vi "Clean Up.vi"(8 "error in (no error)":errorcluster, 11 "PXI in":refnum<class "PXI.lvclass">) -> (0 "error out":errorcluster, 3 "PXI out":refnum<class "PXI.lvclass">)   [LabVIEW 2013, in "PXI.lvclass"]
uses:
  PXI.lvclass
  PXI.lvclass/PXI.ctl
  <resource>/objmgr/daqmx.rc
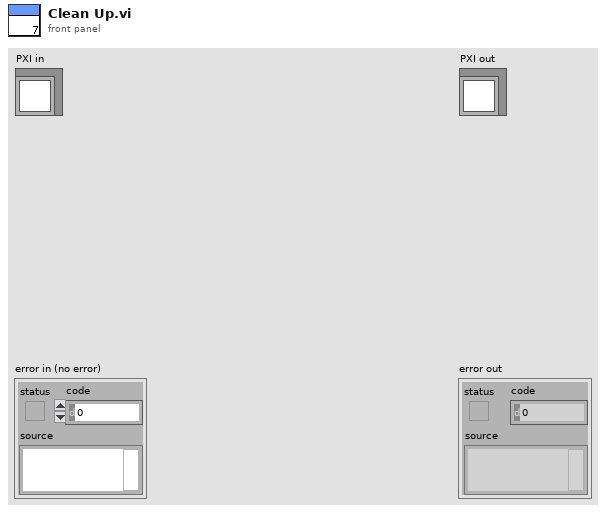
[diagram p1: front panel]
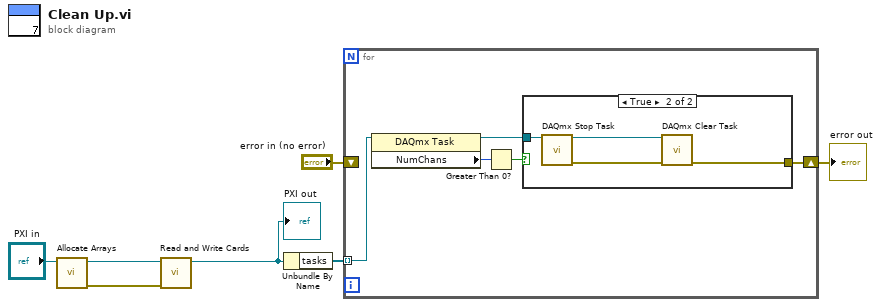
[diagram p0: block diagram]
diagram:
  n1 = call "Allocate Arrays.vi"("PXI in"="PXI in") -> ("error out"=w1:errorcluster, "PXI out"=w5:refnum<class "PXI.lvclass">)  [unwired: 9 in]
  n2 = call "Read and Write Cards.vi"("error in (no error)"=w1, "PXI in"=w5) -> ("PXI out"=w3:refnum<class "PXI.lvclass">)  [unwired: 8 in, 1 out]
  "PXI out" <- w3
  n3 = Unbundle By Name(w3) -> ("tasks"=w6:refnum<k21>[])
  n4 = for {
    tunnel: w6 -> [w8] mode=indexing
    shift-right: [w9] -> w7
    shift-left: "error in (no error)" -> [_]
    n5 = property class="DAQmx Task"(reference=w8) -> (reference out=w10:refnum<k21>, "NumChans"=w12:u32)  [unwired: 1 in, 1 out]
    n6 = Greater Than 0?(x=w12) -> (x > 0?=w11:bool)
    n7 = case shown="True" w11 {
      tunnel: w10 -> [_ w14]
      tunnel: [_ w13] -> w9
      frame False {
      }
      frame True {
        n8 = call <vilib>:"DAQmx Stop Task.vi"("task/channels in"=w14) -> ("task out"=w16:refnum<k21>, "error out"=w15:errorcluster)  [unwired: 13 in]
        n9 = call <vilib>:"DAQmx Clear Task.vi"("task in"=w16, "error in"=w15) -> ("error out"=w13:errorcluster)  [unwired: 13 in]
      }
    }
  }
  "error out" <- w7
